vi "Remove Queue.vi"(9 "Queue":refnum<queue>, 11 "Channel Data In":T1) -> (3 "Channel Data":T1)   [LabVIEW 2020, in "Flex.lvlib"]
uses:
  Flex.lvlib
  Channel Data.ctl
  Element.ctl
  Element Info.ctl
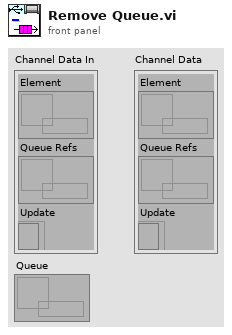
[diagram p1: front panel]
types:
  T1 = typedef "Flex.lvlib/Channel Data.ctl" = cluster{"Element":refnum<data-value>, "Queue Refs":refnum<data-value>, "Update":refnum<k4>}
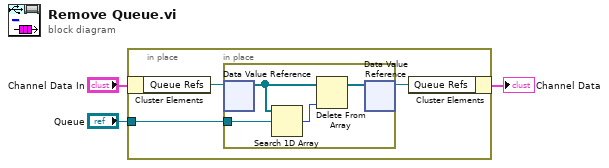
[diagram p0: block diagram]
diagram:
  n1 = in-place {
    in-place-border: "Queue" -> [w4]
    n2 = in-place-cluster #1("Channel Data In") -> ("Queue Refs"=w6:refnum<data-value>)
    n3 = in-place {
      in-place-border: w4 -> [w10]
      n4 = in-place-dvr #2(w6) -> (w9:refnum<queue>[])  [unwired: 1 out]
      n5 = Search 1D Array(1D array=w9, element=w10) -> (index of element=w8:i32)  [unwired: 1 in]
      n6 = Delete From Array(array=w9, index=w8) -> (array with subset deleted=w7:refnum<queue>[])  [unwired: 1 in, 1 out]
      n7 = in-place-dvr #2(w7) -> (w5:refnum<data-value>)  [unwired: 1 out]
    }
    n8 = in-place-cluster #1("Queue Refs"=w5) -> (→"Channel Data":T1)
  }
